vi "Reduced Array.vi"(8 "error in (no error)":errorcluster, 9 "terminal count":u32=50, 10 "RTD":i32, 11 "initialized array in":dbl[][](array[numeric])) -> (0 "error out":errorcluster, 2 "start index":u32, 3 "reduced array out":dbl[][](array[numeric]))   [LabVIEW 2019, in "Zen Analytics.lvlib" / "Zen Analytics.lvclass"]
uses:
  Zen Analytics.lvclass
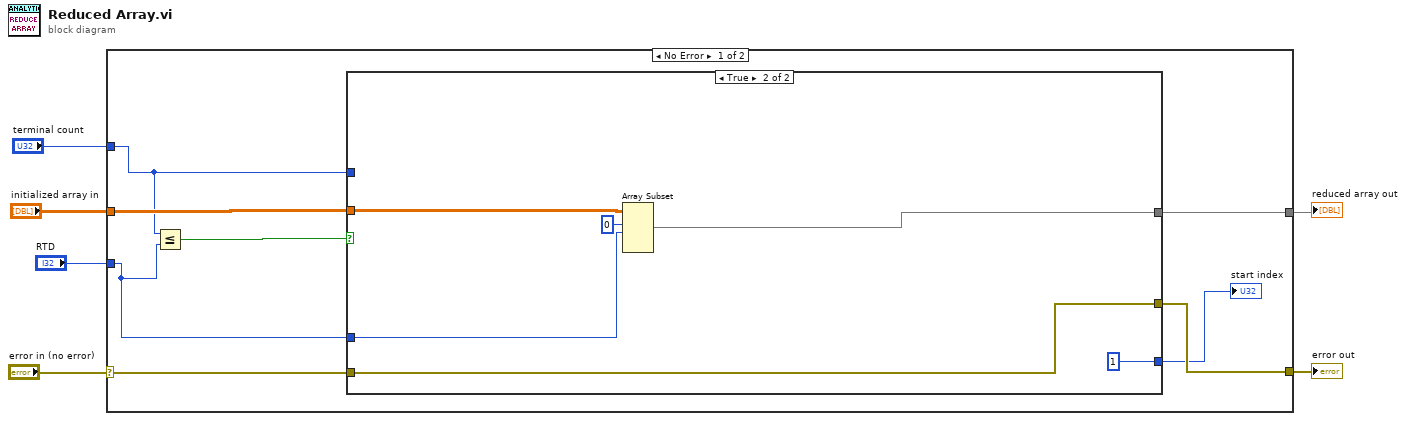
[diagram p0: block diagram]
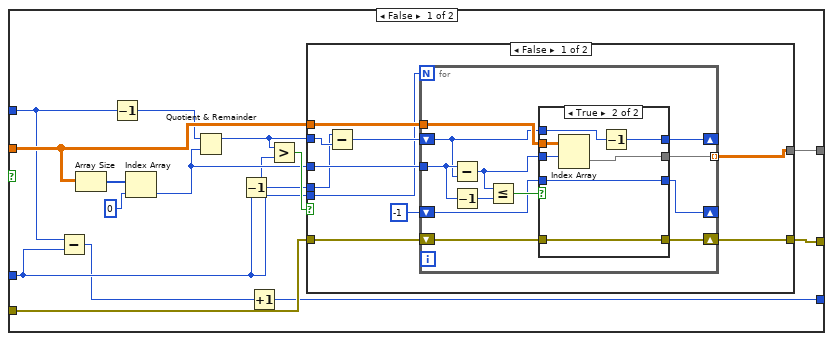
[diagram p2: hidden frame]
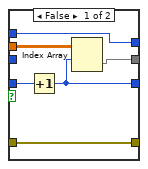
[diagram p3: hidden frame]
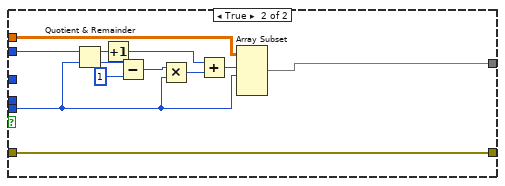
[diagram p4: hidden frame]
diagram:
  n1 = case shown="No Error" "error in (no error)" {
    selector: "error in (no error)" -> [w12 w84]
    tunnel: [w11 w84] -> w1
    tunnel: "initialized array in" -> [w14 w83]
    tunnel: [w13 w83] -> w4
    tunnel: "terminal count" -> [w8 _]
    tunnel: "RTD" -> [w7 _]
    frame No Error {
      n2 = Less Or Equal?(x=w8, y=w7) -> (x <= y?=w9:bool)
      n3 = case shown="True" w9 {
        tunnel: w14 -> [w27 w82]
        tunnel: [w26 w80] -> w13
        tunnel: w12 -> [w22 w79]
        tunnel: [w21 w79] -> w11
        tunnel: [w15 u32 1] -> w10
        tunnel: w8 -> [w20 _]
        tunnel: w7 -> [w18 w77]
        frame False {
          n4 = Subtract(x=w20, y=w18) -> (x-y=w17:u32)
          n5 = Array Size(array=w27) -> (size(s)=w25:i32[])
          n6 = Decrement(x=w20) -> (x-1=w19:u32)
          n7 = Index Array(array=w25, index=0) -> (element=w23:i32)
          n8 = Quotient & Remainder(x=w19, y=w23) -> (x-y*floor(x/y)=w28:u32)  [unwired: 1 out]
          n9 = Decrement(x=w18) -> (x-1=w16:i32)
          n10 = Increment(x=w17) -> (x+1=w15:u32)
          n11 = Greater?(x=w28, y=w16) -> (0:w29:bool)
          n12 = case shown="False" w29 {
            tunnel: w27 -> [w39 w76]
            tunnel: w28 -> [w38 w75]
            tunnel: w18 -> [w31 w66]
            tunnel: w23 -> [w36 _]
            tunnel: [w34 w72] -> w26
            tunnel: w22 -> [w33 w70]
            tunnel: [w32 w70] -> w21
            tunnel: w16 -> [w30 _]
            frame False {
              n13 = Subtract(x=w30, y=w38) -> (x-y=w37:u32)
              n14 = for {
                N: w31 -> [_]
                tunnel: w39 -> [w48]
                tunnel: w36 -> [w51]
                shift-right: [w46] -> _
                shift-left: -1 -> [w47]
                tunnel: [w42] -> w34 mode=indexing
                shift-right: [w44] -> _
                shift-left: w37 -> [w43]
                shift-right: [w41] -> w32
                shift-left: w33 -> [w40]
                n15 = Subtract(x=w51, y=w43) -> (x-y=w45:u32)
                n16 = Decrement(x=w51) -> (x-1=w50:i32)
                n17 = Less Or Equal?(x=w45, y=w50) -> (x <= y?=w49:bool)
                n18 = case shown="True" w49 {
                  tunnel: w48 -> [w56 w64]
                  tunnel: w47 -> [w57 w63]
                  tunnel: [w55 w63] -> w46
                  tunnel: w45 -> [_ w62]
                  tunnel: [w54 w60] -> w44
                  tunnel: w43 -> [w54 w61]
                  tunnel: [w53 w59] -> w42
                  tunnel: [w52 w58] -> w41
                  tunnel: w40 -> [w52 w58]
                  frame False {
                    n19 = Increment(x=w57) -> (x+1=w55:i32)
                    n20 = Index Array "Index Array"(array=w56, index (row)=w55) -> (element=w53:dbl[])  [unwired: 1 in]
                  }
                  frame True {
                    n21 = Index Array "Index Array"(array=w64, index (row)=w62) -> (element=w59:dbl[])  [unwired: 1 in]
                    n22 = Decrement(x=w61) -> (x-1=w60:u32)
                  }
                }
              }
            }
            frame True {
              n23 = Quotient & Remainder(x=w75, y=w66) -> (x-y*floor(x/y)=w74:u32, floor(x/y)=w69:u32)
              n24 = Increment(x=w74) -> (x+1=w65:u32)
              n25 = Subtract(x=w69, y=u32 1) -> (x-y=w67:u32)
              n26 = Multiply(x=w67, y=w66) -> (x*y=w73:u32)
              n27 = Add(x=w65, y=w73) -> (x+y=w71:u32)
              n28 = Array Subset(array=w76, index (row)=w71, length (row)=w66) -> (w72:dbl[][])  [unwired: 2 in]
            }
          }
        }
        frame True {
          n29 = Array Subset(array=w82, index (row)=0 ("index"), length (row)=w77) -> (w80:dbl[][])  [unwired: 2 in]
        }
      }
      "start index" <- w10
    }
    frame Error {
    }
  }
  "error out" <- w1
  "reduced array out" <- w4
